vi "Unit Test.vi"() -> ()   [LabVIEW 2019, in "Andor.lvlib"]
uses:
  Andor.lvlib
  User Event/Controls/UE Abort Action.ctl
panel:
  in  "Expo(s)":dbl format="%#_13g"
  in  "Change Expo":bool
  in  "Grab Stop":bool
  in  "Grab":bool
  in  "Snap":bool
  in  "Open":bool
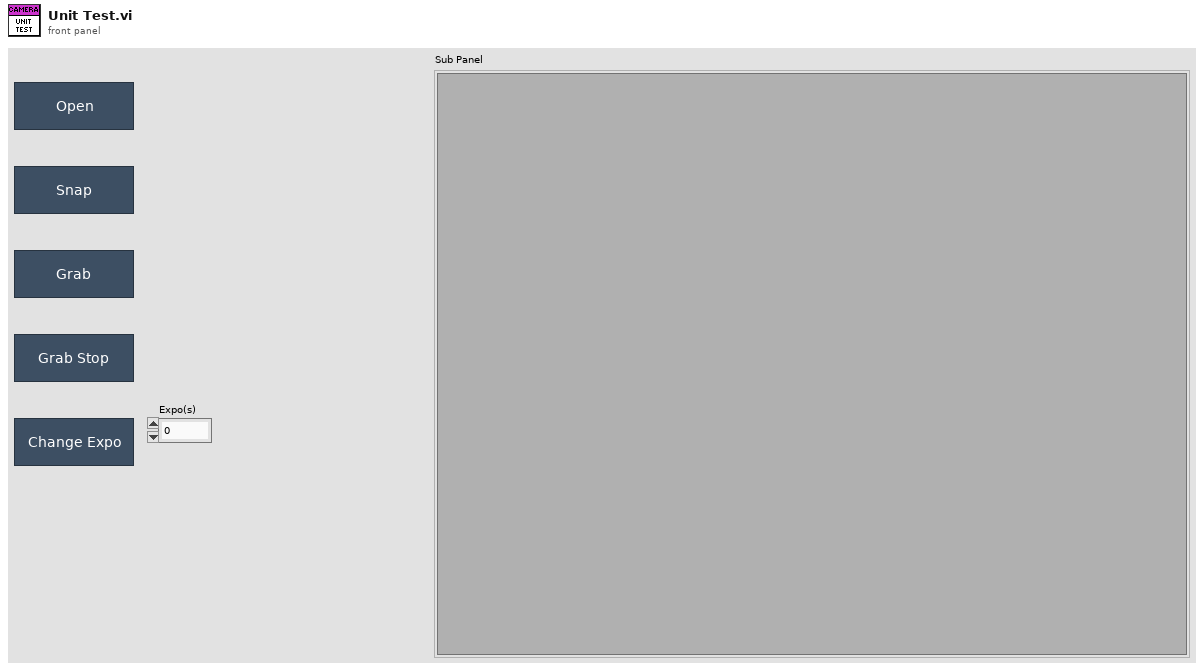
[diagram p1: front panel]
types:
  T1 = typedef "UE Abort Action.ctl" = enum16{"Create", "Get", "Destroy"}
  T2 = typedef "Andor.lvlib/SEQ Data.ctl" = cluster{"Initialize Sucess?":bool, "Image Ref":T3, "VI Refnum":refnum<vi>}
  T3 = typedef "IMAQ Image.ctl" = refnum<image>
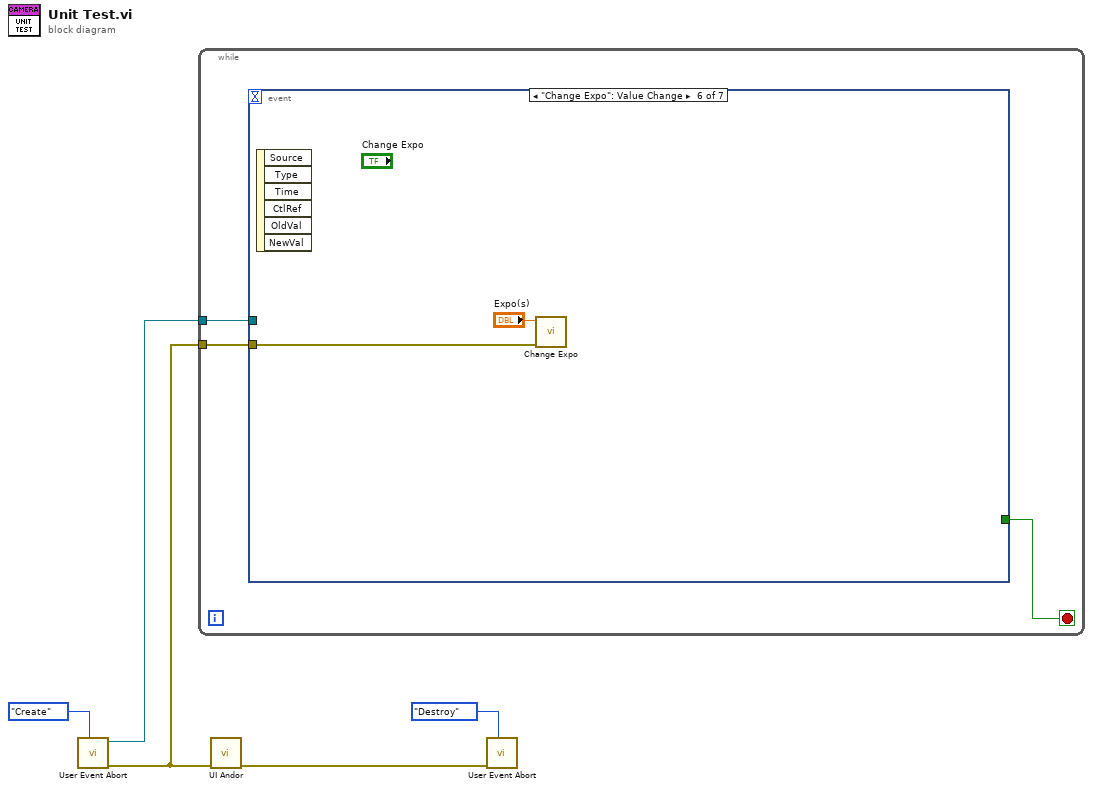
[diagram p0: block diagram]
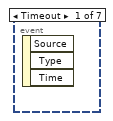
[diagram p2: hidden frame]
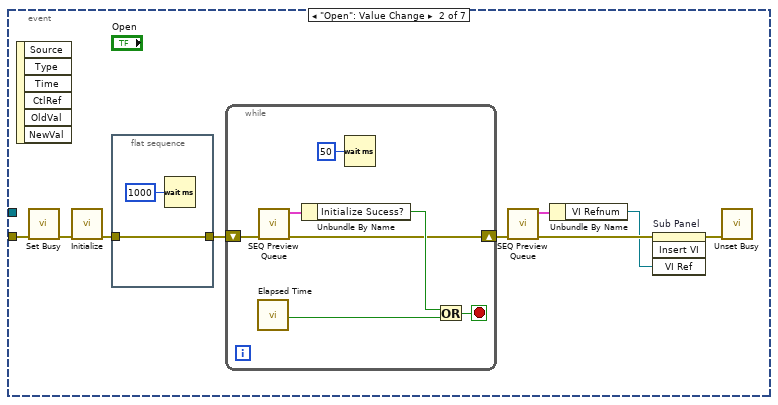
[diagram p3: hidden frame]
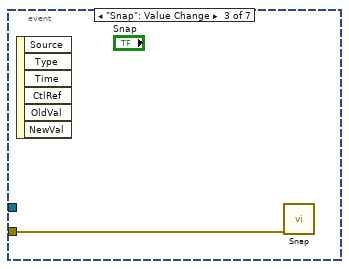
[diagram p4: hidden frame]
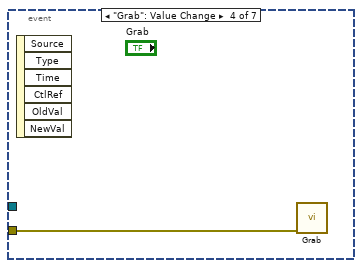
[diagram p5: hidden frame]
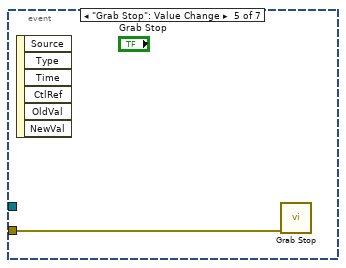
[diagram p6: hidden frame]
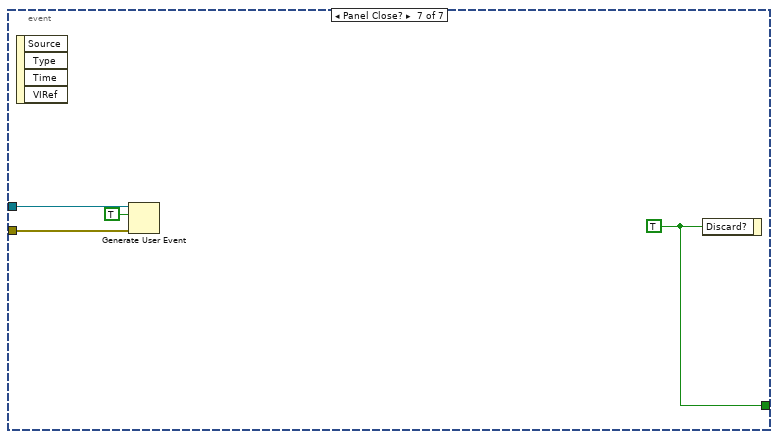
[diagram p7: hidden frame]
diagram:
  n1 = call "User Event Abort.vi"("Action"=UE_Abort_Action."Create") -> ("Error Out"=w1:errorcluster, "User Event Out"=w4:refnum<user-event>)  [unwired: 9 in]
  n2 = while {
    tunnel: w4 -> [w8]
    tunnel: w1 -> [w7]
    stop <- w6 stop-if-true
    n3 = event shown="[5] \"Change Expo\": Value Change" {
      selector: _ -> [_ _ _ _ _ _ _]
      dyn-events: _ -> [_ _ _ _ _ _ _]
      timeout: _ -> [_ _ _ _ _ _ _]
      tunnel: w8 -> [_ _ _ _ _ _ w35]
      tunnel: w7 -> [_ w17 w27 w28 w29 w31 w33]
      tunnel: [_ _ _ _ _ _ w32] -> w6
      event Timeout {
        n4 = event-data() -> ()  [unwired: 1 in, 3 out]
      }
      event "Open": Value Change {
        n5 = event-data() -> ()  [unwired: 1 in, 6 out]
        n6 = call <vilib>:"Set Busy.vi"("error in (no error)"=w17) -> ("error out"=w16:errorcluster)  [unwired: 9 in, 1 out]
        n7 = call "Initialize.vi"("Error In"=w16) -> ("Error Out"=w15:errorcluster)  [unwired: 10 in]
        n8 = flat-sequence {
          tunnel: w15 -> [w25]
          tunnel: [w25] -> w14
          frame #0 {
            n9 = Wait (ms)(milliseconds to wait=u32 1000) -> ()  [unwired: 1 out]
          }
        }
        n10 = while {
          shift-right: [w18] -> w13
          shift-left: w14 -> [w23]
          stop <- w21 stop-if-true
          n11 = call "Elapsed Time"() -> ("Time has Elapsed"=w19:bool)  [unwired: 12 in, 7 out]
          n12 = call "SEQ Preview Queue.vi"("error in"=w23) -> ("error out"=w18:errorcluster, "SEQ Data"=w22:T2)  [unwired: 9 in]
          n13 = Unbundle By Name(w22) -> ("Initialize Sucess?"=w20:bool)
          n14 = Wait (ms)(milliseconds to wait=u32 50) -> ()  [unwired: 1 out]
          n15 = Or(x=w20, y=w19) -> (x .or. y?=w21:bool)
        }
        n16 = call "SEQ Preview Queue.vi"("error in"=w13) -> ("error out"=w11:errorcluster, "SEQ Data"=w12:T2)  [unwired: 9 in]
        n17 = Unbundle By Name(w12) -> ("VI Refnum"=w9:refnum<vi>)
        n18 = invoke on="Sub Panel" class="SubPnl" method="Insert VI"(error in=w11, "VI Ref"=w9) -> (error out=w10:errorcluster)  [unwired: 2 in, 3 out]
        n19 = call <vilib>:"Unset Busy.vi"("error in (no error)"=w10) -> ()  [unwired: 10 in, 1 out]
      }
      event "Snap": Value Change {
        n20 = event-data() -> ()  [unwired: 1 in, 6 out]
        n21 = call "Snap.vi"("Error In"=w27) -> ()  [unwired: 10 in, 1 out]
      }
      event "Grab": Value Change {
        n22 = event-data() -> ()  [unwired: 1 in, 6 out]
        n23 = call "Grab.vi"("Error In"=w28) -> ()  [unwired: 10 in, 1 out]
      }
      event "Grab Stop": Value Change {
        n24 = event-data() -> ()  [unwired: 1 in, 6 out]
        n25 = call "Grab Stop.vi"("Error In"=w29) -> ()  [unwired: 10 in, 1 out]
      }
      event "Change Expo": Value Change {
        n26 = event-data() -> ()  [unwired: 1 in, 6 out]
        n27 = call "Change Expo.vi"("Error In"=w31, "Expo(s)"="Expo(s)") -> ()  [unwired: 9 in, 1 out]
      }
      event Panel Close? {
        w32 = TRUE ("Discard?")
        n28 = event-data() -> ()  [unwired: 1 in, 4 out]
        n29 = Generate User Event(user event=w35, event data cluster=TRUE ("event data"), error in=w33) -> ()  [unwired: 1 in, 2 out]
        n30 = event-data("Discard?"=w32) -> ()  [unwired: 1 in, 1 out]
      }
    }
  }
  n31 = call "UI Andor.vi"("error in"=w1) -> ("error out"=w5:errorcluster)  [unwired: 10 in]
  n32 = call "User Event Abort.vi"("Action"=UE_Abort_Action."Destroy", "Error In"=w5) -> ()  [unwired: 8 in, 2 out]
